vi "HT_multiply.vi"(8 "input valid":bool=TRUE, 10 "y":fxp<+/-,16,2>, 11 "x":fxp<+/-,16,14>) -> (0 "output valid":bool, 3 "x*y":fxp<+/-,16,14>)   [LabVIEW 2013]
uses:
  <vilib>/rvi/FXPMathLib/FxpConvert/subVIs/nifxpmath_Convert_SimConfig.ctl
  <vilib>/fxp/LVFixedPointQuantizationPolicyTypeDef.ctl
  <vilib>/fxp/LVFixedPointOverflowPolicyTypeDef.ctl
  <vilib>/rvi/FXPMathLib/FxpConvert/simVIs/DllFxpConvertTemp_sub.vi
  <vilib>/rvi/FXPMathLib/FxpConvert/XNode/nifxpmath_Convert.xnode
  <vilib>/rvi/FXPMathLib/FxpMul/XNode/nifxpmath_Multiplier.xnode
  <vilib>/rvi/FXPMathLib/FxpInterpret/XNode/nifxpmath_Interpret.xnode
  <vilib>/rvi/FXPMathLib/sim/FxpSim.dll
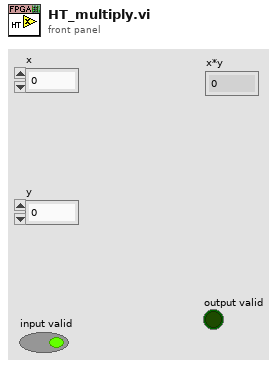
[diagram p1: front panel]
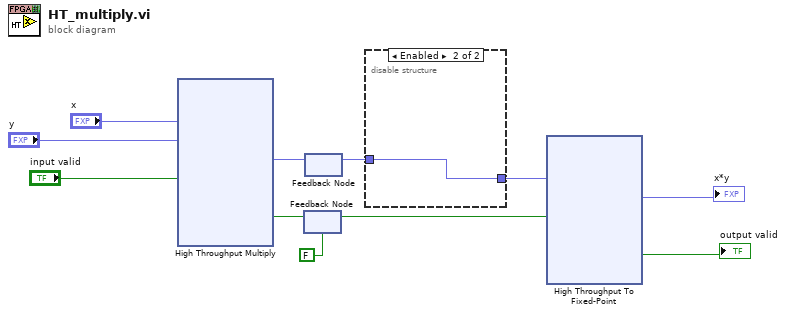
[diagram p0: block diagram]
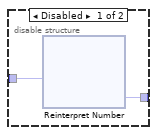
[diagram p2: hidden frame]
diagram:
  n1 = xnode ("High Throughput Multiply")("x"="x", "y"="y", "input valid"="input valid") -> ("x*y"=w11:fxp<+/-,32,16>, "output valid"=w10:bool)  [unwired: 1 in, 1 out]
  n2 = feedback #1(FALSE ("output valid")) -> (w5:bool)
  n3 = feedback-in #1(w10) -> ()
  n4 = feedback #2() -> (w2:fxp<+/-,32,16>)  [unwired: 1 in]
  n5 = feedback-in #2(w11) -> ()
  n6 = disable-structure shown="Enabled" {
    disable-tunnel: w2 -> [w13 w14]
    disable-tunnel: [w12 w14] -> w1
    frame Disabled {
      n7 = xnode "Reinterpret Number"("x"=w13) -> ("y"=w12:fxp<+/-,32,16>)
    }
    frame Enabled {
    }
  }
  n8 = xnode "High Throughput To Fixed-Point"("x"=w1, "input valid"=w5) -> ("y"=→"x*y":fxp<+/-,16,14>, "output valid"=→"output valid":bool)  [unwired: 1 in, 1 out]
